vi "5_4.vi"() -> ()   [LabVIEW 2015]
panel:
  in  "Stop Button":bool
  in  "Save":bool caption="Blank Button"
  in  "Open":bool caption="Blank Button"
  in  "New":bool caption="Blank Button"
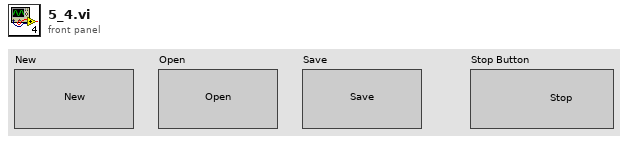
[diagram p1: front panel]
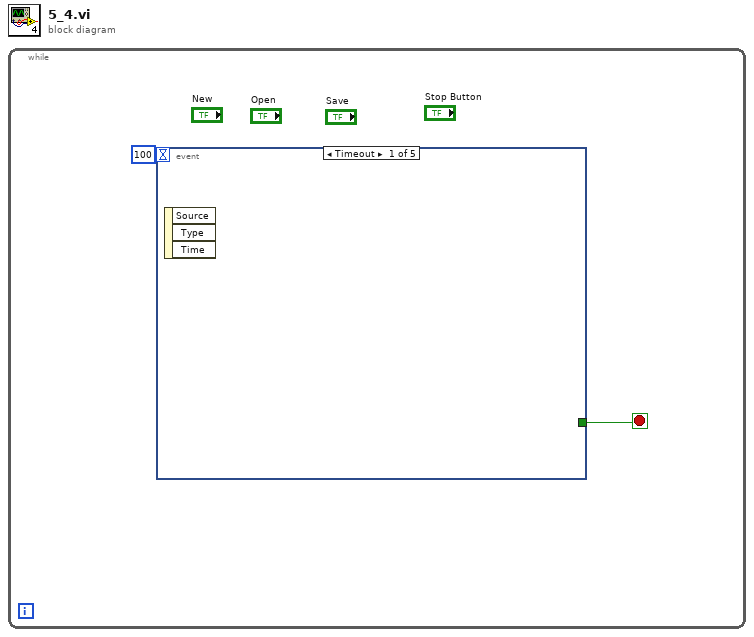
[diagram p0: block diagram]
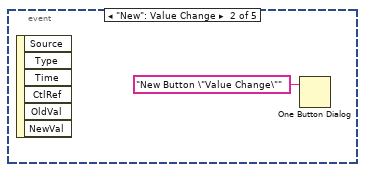
[diagram p2: hidden frame]
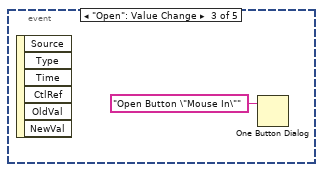
[diagram p3: hidden frame]
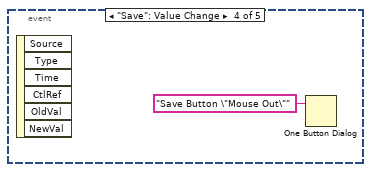
[diagram p4: hidden frame]
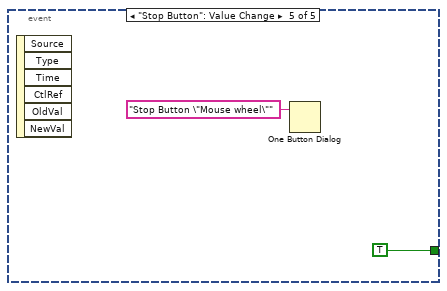
[diagram p5: hidden frame]
diagram:
  n1 = while {
    stop <- w1 stop-if-true
    n2 = event shown="[0] Timeout" {
      selector: _ -> [_ _ _ _ _]
      dyn-events: _ -> [_ _ _ _ _]
      timeout: 100 -> [_ _ _ _ _]
      tunnel: [_ _ _ _ TRUE] -> w1
      event Timeout {
        n3 = event-data() -> ()  [unwired: 1 in, 3 out]
      }
      event "New": Value Change {
        n4 = event-data() -> ()  [unwired: 1 in, 6 out]
        n5 = One Button Dialog(message="New Button \"Value Change\"") -> ()  [unwired: 1 in, 1 out]
      }
      event "Open": Value Change {
        n6 = event-data() -> ()  [unwired: 1 in, 6 out]
        n7 = One Button Dialog(message="Open Button \"Mouse In\"") -> ()  [unwired: 1 in, 1 out]
      }
      event "Save": Value Change {
        n8 = event-data() -> ()  [unwired: 1 in, 6 out]
        n9 = One Button Dialog(message="Save Button \"Mouse Out\"") -> ()  [unwired: 1 in, 1 out]
      }
      event "Stop Button": Value Change {
        n10 = event-data() -> ()  [unwired: 1 in, 6 out]
        n11 = One Button Dialog(message="Stop Button \"Mouse wheel\"") -> ()  [unwired: 1 in, 1 out]
      }
    }
  }
